vi "Simple Array - Failure Message.vi"() -> ()   [LabVIEW 2017, in "Transparent Assertions.Tests.lvlib" / "Assert Collection Not Contains.lvlib"]
uses:
  Assert Collection Not Contains.lvlib
  src/Transparent Assertions/Transparent Assertions.lvlib
panel:
  out "error out":errorcluster
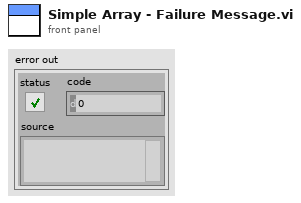
[diagram p1: front panel]
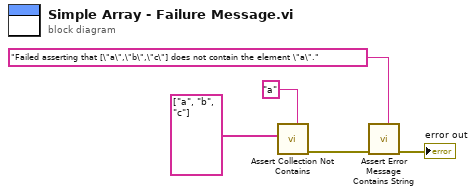
[diagram p0: block diagram]
diagram:
  n1 = call "Assert Collection Not Contains.vi"("Expected"="a", "Collection"=string[] ["a", "b", "c"]) -> ("error out"=w1:errorcluster)  [unwired: 9 in]
  n2 = call "Assert Error Message Contains String.vi"("Expected"="Failed asserting that [\"a\",\"b\",\"c\"] does not contain the element \"a\".", "error in (no error)"=w1) -> ("error out"=→"error out":errorcluster)  [unwired: 9 in]
